vi "Read Part.vi"(8 "error in (no error)":errorcluster, 11 "Multipart Parser in":refnum<class "Multipart Parser.lvclass">) -> (0 "error out":errorcluster, 3 "Multipart Parser out":refnum<class "Multipart Parser.lvclass">, 4 "Last?":bool)   [LabVIEW 2020, in "HTTP Utils.lvlib" / "Multipart Parser.lvclass"]
uses:
  Multipart Parser.lvclass
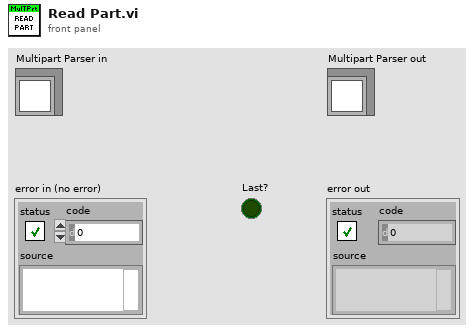
[diagram p1: front panel]
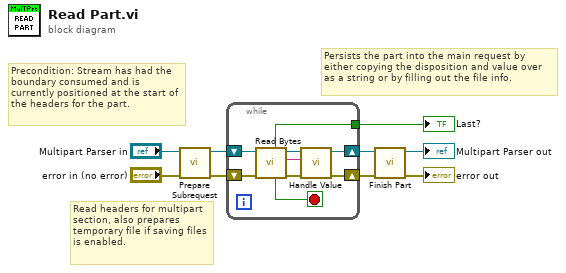
[diagram p0: block diagram]
diagram:
  # "Persists the part into the main request by either copying the disposition and value over as a string or by filling out the file info."
  # "Read headers for multipart section, also prepares temporary file if saving files is enabled."
  # "Precondition: Stream has had the boundary consumed and is currently positioned at the start of the headers for the part."
  n1 = call "Prepare Subrequest.vi"("error in (no error)"="error in (no error)", "Multipart Parser in"="Multipart Parser in") -> ("error out"=w6:errorcluster, "Multipart Parser out"=w7:refnum<class "Multipart Parser.lvclass">)  [unwired: 8 in]
  n2 = while {
    shift-right: [w12] -> w4
    shift-left: w7 -> [w18]
    shift-right: [w11] -> w3
    shift-left: w6 -> [w17]
    tunnel: [w10] -> w5
    stop <- w13 stop-if-true
    n3 = call "Read Bytes.vi"("error in (no error)"=w17, "Multipart Parser in"=w18) -> ("error out"=w14:errorcluster, "Value"=w15:string, "Multipart Parser out"=w16:refnum<class "Multipart Parser.lvclass">, "Boundary"=w13:bool, "Last"=w10:bool)  [unwired: 5 in]
    n4 = call "Handle Value.vi"("error in (no error)"=w14, "Value"=w15, "Multipart Parser in"=w16) -> ("error out"=w11:errorcluster, "Multipart Parser out"=w12:refnum<class "Multipart Parser.lvclass">)  [unwired: 7 in]
  }
  "Last?" <- w5
  n5 = call "Finish Part.vi"("error in (no error)"=w3, "Multipart Parser in"=w4) -> ("error out"=→"error out":errorcluster, "Multipart Parser out"=→"Multipart Parser out":refnum<class "Multipart Parser.lvclass">)  [unwired: 8 in]
